vi "Timer.vi"(3 "Reset":bool, 4 "Delay":u32, 5 "Name":string) -> (0 "Running":bool, 1 "End Trigger":bool, 2 "Start Trigger":bool)   [LabVIEW 2012, in "femtoRoboLib.lvlib"]
doc: "Create/update a Timer. After Timer is already running, Delay does nothing. Remember to Reset before reusing a named Timer. Has triggers for the beginning and end of the time period."
uses:
  femtoRoboLib.lvlib
panel:
  in  "Timers":u32[](array[numeric])
  in  "Names":string[](array[string])
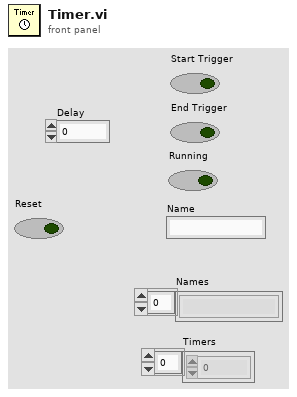
[diagram p1: front panel]
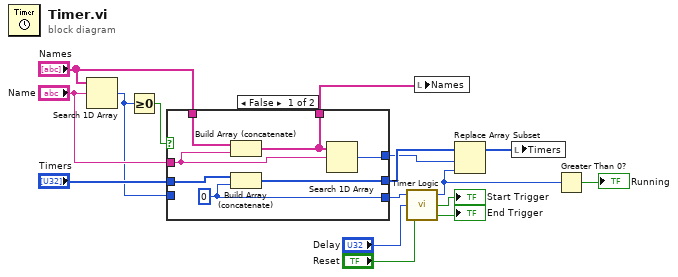
[diagram p0: block diagram]
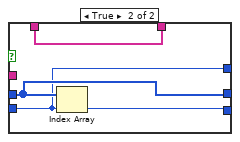
[diagram p2: hidden frame]
diagram:
  n1 = Search 1D Array(1D array="Names", element="Name") -> (index of element=w3:i32)  [unwired: 1 in]
  n2 = Greater Or Equal To 0?(x=w3) -> (x >= 0?=w15:bool)
  n3 = case shown="False" w15 {
    tunnel: w3 -> [_ w24]
    tunnel: [w21 w27] -> w16
    tunnel: "Timers" -> [w22 w25]
    tunnel: "Names" -> [w23 w26]
    tunnel: "Name" -> [w17 _]
    tunnel: [w19 w26] -> w12
    tunnel: [w20 w25] -> w11
    tunnel: [w18 w24] -> w10
    frame False {
      w21 = u32 0
      n4 = Build Array (concatenate)(w23, w17) -> (w19:string[])
      n5 = Build Array (concatenate)(w22, w21) -> (w20:u32[])
      n6 = Search 1D Array(1D array=w19, element=w17) -> (index of element=w18:i32)  [unwired: 1 in]
    }
    frame True {
      n7 = Index Array(array=w25, index=w24) -> (element=w27:u32)
    }
  }
  n8 = call "Timer Logic.vi"("Reset"="Reset", "Delay"="Delay", "Timer In"=w16) -> ("End Trigger"=→"End Trigger":bool, "Start Trigger"=→"Start Trigger":bool, "Timer Out"=w1:u32)
  n9 = local write "Names"(w12) -> ()
  n10 = Replace Array Subset(array=w11, new element=w1, index=w10) -> (w9:u32[])
  n11 = local write "Timers"(w9) -> ()
  n12 = Greater Than 0?(x=w1) -> (x > 0?=→"Running":bool)
